vi "BoP Output Read Client.vi"() -> ()   [LabVIEW 2017]
uses:
  <vilib>/OPCUA/controls/NodeIds.ctl
  <vilib>/OPCUA/controls/NodeId.ctl
  <vilib>/OPCUA/NI OPC UA Client.lvlib
panel:
  in  "stop":bool
  out "error out":errorcluster
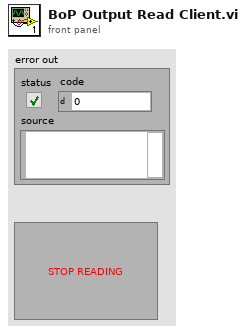
[diagram p1: front panel]
types:
  T1 = cluster{"message mode":enum16{"None", "Sign", "Sign and Encrypt"}, "security":enum16{"Basic256", "Basic128Rsa15"}}
  T2 = typedef "NodeIds.ctl" = T3[]
  T3 = typedef "NodeId.ctl" = string
  T4 = typedef "OPC UA Client Refnum.ctl" = refnum<k21>
  T5 = typedef "Subscription ID.ctl" = u32
  T6 = typedef "Subscription Data Change.ctl" = cluster{"node ID":T3, " value":variant, "timestamp":timestamp, "data type":T7, "status code":T8}
  T7 = typedef "Data Type.ctl" = u16
  T8 = typedef "OPC UA StatusCode.ctl" = u32
  T9 = cluster{"[0]":sgl, "[1]":sgl, "[2]":sgl, "[3]":sgl, "[4]":sgl, "[5]":sgl, "[6]":sgl, "[7]":sgl, "[8]":sgl, "[9]":sgl, "[10]":sgl, "[11]":sgl, "[12]":sgl, "[13]":sgl, "[14]":sgl, "[15]":sgl, "[16]":sgl, "[17]":sgl, "[18]":sgl, "[19]":sgl, "[20]":sgl, "[21]":sgl, "[22]":sgl, "[23]":sgl, "[24]":sgl, "[25]":sgl, "[26]":sgl, "[27]":sgl, "[28]":sgl, "[29]":sgl}
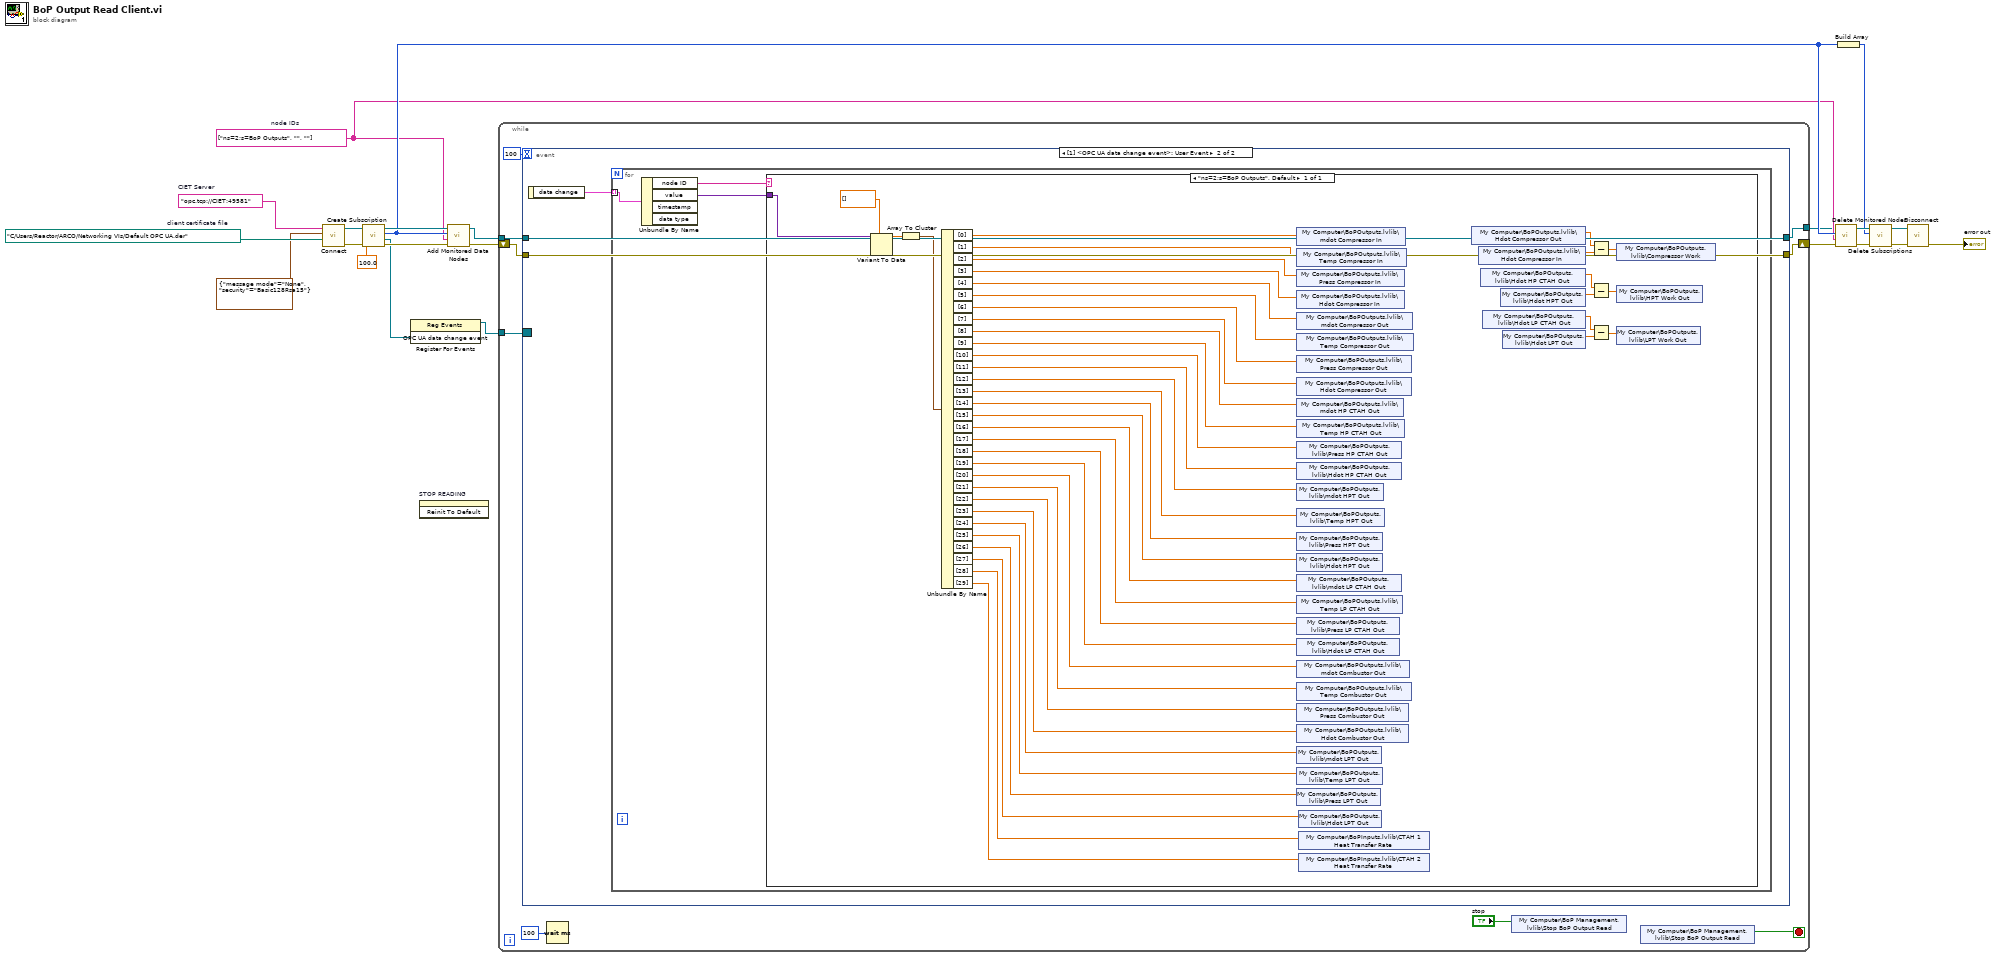
[diagram p0: block diagram]
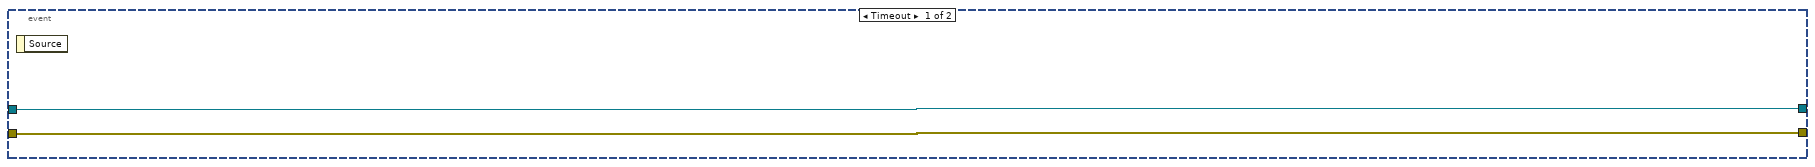
[diagram p2: hidden frame]
diagram:
  w5 = T2 ["ns=2;s=BoP Outputs", "", ""]  # node IDs
  w20 = path "C:/Users/Reactor/ARCO/Networking VIs/Default OPC UA.der"  # client certificate file
  w21 = "opc.tcp://CIET:49581"  # CIET Server
  n1 = call <vilib>:"Connect.vi"("client certificate file"=w20, "security policy"=T1 {"message mode"=enum."None", "security"=enum."Basic128Rsa15"}, "server endpoint URL"=w21) -> ("error out"=w2:errorcluster, "OPC UA client refnum out"=w18:T4)  [unwired: 6 in, 1 out]
  n2 = call <vilib>:"Create Subscription.vi"("error in (no error)"=w2, "publishing interval (1000 ms)"=100.0, "OPC UA client refnum in"=w18) -> ("error out"=w16:errorcluster, "OPC UA data change event"=w15:refnum<user-event>, "subscription ID out"=w10:T5, "OPC UA client refnum out"=w17:T4)  [unwired: 4 in, 1 out]
  n3 = register-events(w15) -> (reference out=w8:refnum<event-registration>)  [unwired: 2 in, 1 out]
  n4 = invoke on="STOP READING" class="Bool" method="Reinit To Default"() -> ()  [unwired: 3 in, 3 out]
  n5 = call <vilib>:"Add Monitored Data Nodes.vi"("error in (no error)"=w16, "node IDs"=w5, "subscription ID in"=w10, "OPC UA client refnum in"=w17) -> ("error out"=w6:errorcluster, "OPC UA client refnum out"=w7:T4)  [unwired: 4 in, 2 out]
  n6 = while {
    tunnel: w8 -> [w31]
    tunnel: w7 -> [w30]
    tunnel: [w29] -> w4
    shift-right: [w27] -> w1
    shift-left: w6 -> [w26]
    stop <- w24 stop-if-true
    n7 = event shown="[1] <OPC UA data change event>: User Event" {
      selector: w31 -> [_ _]
      dyn-events: _ -> [_ _]
      timeout: 100 -> [_ _]
      tunnel: w30 -> [w33 w36]
      tunnel: [w33 w36] -> w29
      tunnel: w26 -> [w32 w35]
      tunnel: [w32 w35] -> w27
      event Timeout {
        n8 = event-data() -> ()  [unwired: 1 in, 1 out]
      }
      event User Event {
        n9 = event-data() -> ("data change"=w34:T6[])  [unwired: 1 in]
        n10 = for {
          tunnel: w34 -> [w39] mode=indexing
          n11 = Unbundle By Name(w39) -> ("node ID"=w38:T3, "value"=w37:variant)  [unwired: 2 out]
          n12 = case shown="\"ns=2;s=BoP Outputs\", Default" w38 {
            tunnel: w37 -> [w82]
            frame "ns=2;s=BoP Outputs", Default {
              n13 = Variant To Data(type=sgl[] [], Variant=w82) -> (data=w80:sgl[])  [unwired: 1 in, 1 out]
              n14 = Array To Cluster(array=w80) -> (cluster=w79:T9)
              n15 = Unbundle By Name(w79) -> ("[0]"=w78:sgl, "[1]"=w77:sgl, "[2]"=w76:sgl, "[3]"=w75:sgl, "[4]"=w74:sgl, "[5]"=w73:sgl, "[6]"=w72:sgl, "[7]"=w71:sgl, "[8]"=w70:sgl, "[9]"=w69:sgl, "[10]"=w68:sgl, "[11]"=w67:sgl, "[12]"=w66:sgl, "[13]"=w65:sgl, "[14]"=w64:sgl, "[15]"=w63:sgl, "[16]"=w62:sgl, "[17]"=w61:sgl, "[18]"=w60:sgl, "[19]"=w59:sgl, "[20]"=w58:sgl, "[21]"=w57:sgl, "[22]"=w56:sgl, "[23]"=w55:sgl, "[24]"=w54:sgl, "[25]"=w53:sgl, "[26]"=w52:sgl, "[27]"=w51:sgl, "[28]"=w41:sgl, "[29]"=w40:sgl)
              n16 = shared-variable "My Computer\\BoPOutputs.lvlib\\mdot Compressor In"(w78) -> ()  [unwired: 1 in, 1 out]
              n17 = shared-variable "My Computer\\BoPOutputs.lvlib\\Temp Compressor In"(w77) -> ()  [unwired: 1 in, 1 out]
              n18 = shared-variable "My Computer\\BoPOutputs.lvlib\\Press Compressor In"(w76) -> ()  [unwired: 1 in, 1 out]
              n19 = shared-variable "My Computer\\BoPOutputs.lvlib\\Hdot Compressor In"(w75) -> ()  [unwired: 1 in, 1 out]
              n20 = shared-variable "My Computer\\BoPOutputs.lvlib\\mdot Compressor Out"(w74) -> ()  [unwired: 1 in, 1 out]
              n21 = shared-variable "My Computer\\BoPOutputs.lvlib\\Temp Compressor Out"(w73) -> ()  [unwired: 1 in, 1 out]
              n22 = shared-variable "My Computer\\BoPOutputs.lvlib\\Press Compressor Out"(w72) -> ()  [unwired: 1 in, 1 out]
              n23 = shared-variable "My Computer\\BoPOutputs.lvlib\\Hdot Compressor Out"(w71) -> ()  [unwired: 1 in, 1 out]
              n24 = shared-variable "My Computer\\BoPOutputs.lvlib\\mdot HP CTAH Out"(w70) -> ()  [unwired: 1 in, 1 out]
              n25 = shared-variable "My Computer\\BoPOutputs.lvlib\\Temp HP CTAH Out"(w69) -> ()  [unwired: 1 in, 1 out]
              n26 = shared-variable "My Computer\\BoPOutputs.lvlib\\Press HP CTAH Out"(w68) -> ()  [unwired: 1 in, 1 out]
              n27 = shared-variable "My Computer\\BoPOutputs.lvlib\\Hdot HP CTAH Out"(w67) -> ()  [unwired: 1 in, 1 out]
              n28 = shared-variable "My Computer\\BoPOutputs.lvlib\\mdot HPT Out"(w66) -> ()  [unwired: 1 in, 1 out]
              n29 = shared-variable "My Computer\\BoPOutputs.lvlib\\Temp HPT Out"(w65) -> ()  [unwired: 1 in, 1 out]
              n30 = shared-variable "My Computer\\BoPOutputs.lvlib\\Press HPT Out"(w64) -> ()  [unwired: 1 in, 1 out]
              n31 = shared-variable "My Computer\\BoPOutputs.lvlib\\Hdot HPT Out"(w63) -> ()  [unwired: 1 in, 1 out]
              n32 = shared-variable "My Computer\\BoPOutputs.lvlib\\mdot LP CTAH Out"(w62) -> ()  [unwired: 1 in, 1 out]
              n33 = shared-variable "My Computer\\BoPOutputs.lvlib\\Temp LP CTAH Out"(w61) -> ()  [unwired: 1 in, 1 out]
              n34 = shared-variable "My Computer\\BoPOutputs.lvlib\\Press LP CTAH Out"(w60) -> ()  [unwired: 1 in, 1 out]
              n35 = shared-variable "My Computer\\BoPOutputs.lvlib\\Hdot LP CTAH Out"(w59) -> ()  [unwired: 1 in, 1 out]
              n36 = shared-variable "My Computer\\BoPOutputs.lvlib\\mdot Combustor Out"(w58) -> ()  [unwired: 1 in, 1 out]
              n37 = shared-variable "My Computer\\BoPOutputs.lvlib\\Temp Combustor Out"(w57) -> ()  [unwired: 1 in, 1 out]
              n38 = shared-variable "My Computer\\BoPOutputs.lvlib\\Press Combustor Out"(w56) -> ()  [unwired: 1 in, 1 out]
              n39 = shared-variable "My Computer\\BoPOutputs.lvlib\\Hdot Combustor Out"(w55) -> ()  [unwired: 1 in, 1 out]
              n40 = shared-variable "My Computer\\BoPOutputs.lvlib\\mdot LPT Out"(w54) -> ()  [unwired: 1 in, 1 out]
              n41 = shared-variable "My Computer\\BoPOutputs.lvlib\\Temp LPT Out"(w53) -> ()  [unwired: 1 in, 1 out]
              n42 = shared-variable "My Computer\\BoPOutputs.lvlib\\Press LPT Out"(w52) -> ()  [unwired: 1 in, 1 out]
              n43 = shared-variable "My Computer\\BoPOutputs.lvlib\\Hdot LPT Out"(w51) -> ()  [unwired: 1 in, 1 out]
              n44 = shared-variable "My Computer\\BoPInputs.lvlib\\CTAH 1 Heat Transfer Rate"(w41) -> ()  [unwired: 1 in, 1 out]
              n45 = shared-variable "My Computer\\BoPInputs.lvlib\\CTAH 2 Heat Transfer Rate"(w40) -> ()  [unwired: 1 in, 1 out]
              n46 = shared-variable "My Computer\\BoPOutputs.lvlib\\Hdot Compressor Out"() -> (w50:sgl)  [unwired: 1 in, 1 out]
              n47 = shared-variable "My Computer\\BoPOutputs.lvlib\\Hdot Compressor In"() -> (w49:sgl)  [unwired: 1 in, 1 out]
              n48 = shared-variable "My Computer\\BoPOutputs.lvlib\\Hdot HP CTAH Out"() -> (w45:sgl)  [unwired: 1 in, 1 out]
              n49 = shared-variable "My Computer\\BoPOutputs.lvlib\\Hdot LP CTAH Out"() -> (w44:sgl)  [unwired: 1 in, 1 out]
              n50 = shared-variable "My Computer\\BoPOutputs.lvlib\\Hdot HPT Out"() -> (w47:sgl)  [unwired: 1 in, 1 out]
              n51 = shared-variable "My Computer\\BoPOutputs.lvlib\\Hdot LPT Out"() -> (w43:sgl)  [unwired: 1 in, 1 out]
              n52 = Subtract(x=w50, y=w49) -> (x-y=w48:sgl)
              n53 = Subtract(x=w45, y=w47) -> (x-y=w46:sgl)
              n54 = Subtract(x=w44, y=w43) -> (x-y=w42:sgl)
              n55 = shared-variable "My Computer\\BoPOutputs.lvlib\\Compressor Work"(w48) -> ()  [unwired: 1 in, 1 out]
              n56 = shared-variable "My Computer\\BoPOutputs.lvlib\\HPT Work Out"(w46) -> ()  [unwired: 1 in, 1 out]
              n57 = shared-variable "My Computer\\BoPOutputs.lvlib\\LPT Work Out"(w42) -> ()  [unwired: 1 in, 1 out]
            }
          }
        }
      }
    }
    n58 = Wait (ms)(milliseconds to wait=u32 100 ("millisecond timer value")) -> ()  [unwired: 1 out]
    n59 = shared-variable "My Computer\\BoP Management.lvlib\\Stop BoP Output Read"("stop") -> ()  [unwired: 1 in, 1 out]
    n60 = shared-variable "My Computer\\BoP Management.lvlib\\Stop BoP Output Read"() -> (w24:bool)  [unwired: 1 in, 1 out]
  }
  n61 = call <vilib>:"Delete Monitored Nodes.vi"("error in (no error)"=w1, "node IDs"=w5, "subscription ID in"=w10, "OPC UA client refnum in"=w4) -> ("error out"=w11:errorcluster, "OPC UA client refnum out"=w12:T4)  [unwired: 3 in, 3 out]
  n62 = Build Array(w10) -> (w9:T5[])
  n63 = call <vilib>:"Delete Subscriptions.vi"("error in (no error)"=w11, "subscription IDs"=w9, "OPC UA client refnum in"=w12) -> ("error out"=w13:errorcluster, "OPC UA client refnum out"=w14:T4)  [unwired: 6 in, 1 out]
  n64 = call <vilib>:"Disconnect.vi"("error in (no error)"=w13, "OPC UA client refnum in"=w14) -> ("error out"=→"error out":errorcluster)  [unwired: 9 in]
